vi "ReadTriggerNode.vi"(8 "Error In":errorcluster, 11 "Multiplexer Node In":refnum<k20>) -> (0 "Error Out":errorcluster, 2 "Trigger Configuration":T1={"Arm"={"Source"=enum."Hold", "Count"=1, "Infinite?"=FALSE}, "Scan"={"Source"=enum."Hold", "Count"=0, "Infinite?"=FALSE, "Delay (sec)"=0.0, "Interval (sec)"=0.0}, "Channel"={"Source"=enum."Hold", "Count"=0, "Infinite?"=FALSE, "Auto Count?"=FALSE, "Delay (sec)"=0.0, "Interval (sec)"=0.0}} {"Arm"."Count" min=1 max=99999 step=1}, 3 "Multiplexer Node Out":refnum<k20>)   [LabVIEW 2012]
uses:
  TriggerConfiguration.ctl
  TriggerArmConfiguration.ctl
  driver/Public/Controls/ArmSource.ctl
  TriggerScanConfiguration.ctl
  driver/Public/Controls/ScanSource.ctl
  TriggerChannelConfiguration.ctl
  driver/Public/Controls/TriggerSource.ctl
  driver/Keithley-7001.lvlib
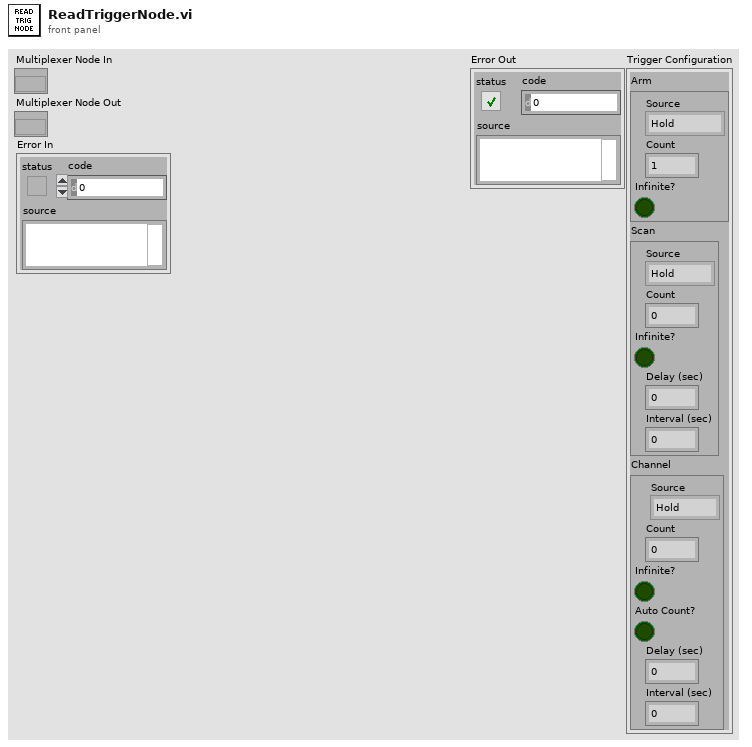
[diagram p1: front panel]
types:
  T1 = typedef "TriggerConfiguration.ctl" = cluster{"Arm":T2, "Scan":T4, "Channel":T6}
  T2 = typedef "TriggerArmConfiguration.ctl" = cluster{"Source":T3, "Count":u32, "Infinite?":bool}
  T3 = typedef "Keithley-7001.lvlib/ArmSource.ctl" = enum16{"Hold", "Immediate", "Manual", "Bus", "TLink", "External"}
  T4 = typedef "TriggerScanConfiguration.ctl" = cluster{"Source":T5, "Count":u32, "Infinite?":bool, "Delay (sec)":dbl, "Interval (sec)":dbl}
  T5 = typedef "Keithley-7001.lvlib/ScanSource.ctl" = enum16{"Hold", "Immediate", "Timer", "Manual", "Bus", "TLink", "External"}
  T6 = typedef "TriggerChannelConfiguration.ctl" = cluster{"Source":T7, "Count":u32, "Infinite?":bool, "Auto Count?":bool, "Delay (sec)":dbl, "Interval (sec)":dbl}
  T7 = typedef "Keithley-7001.lvlib/TriggerSource.ctl" = enum16{"Hold", "Immediate", "Manual", "Bus", "TLink", "External", "Timer"}
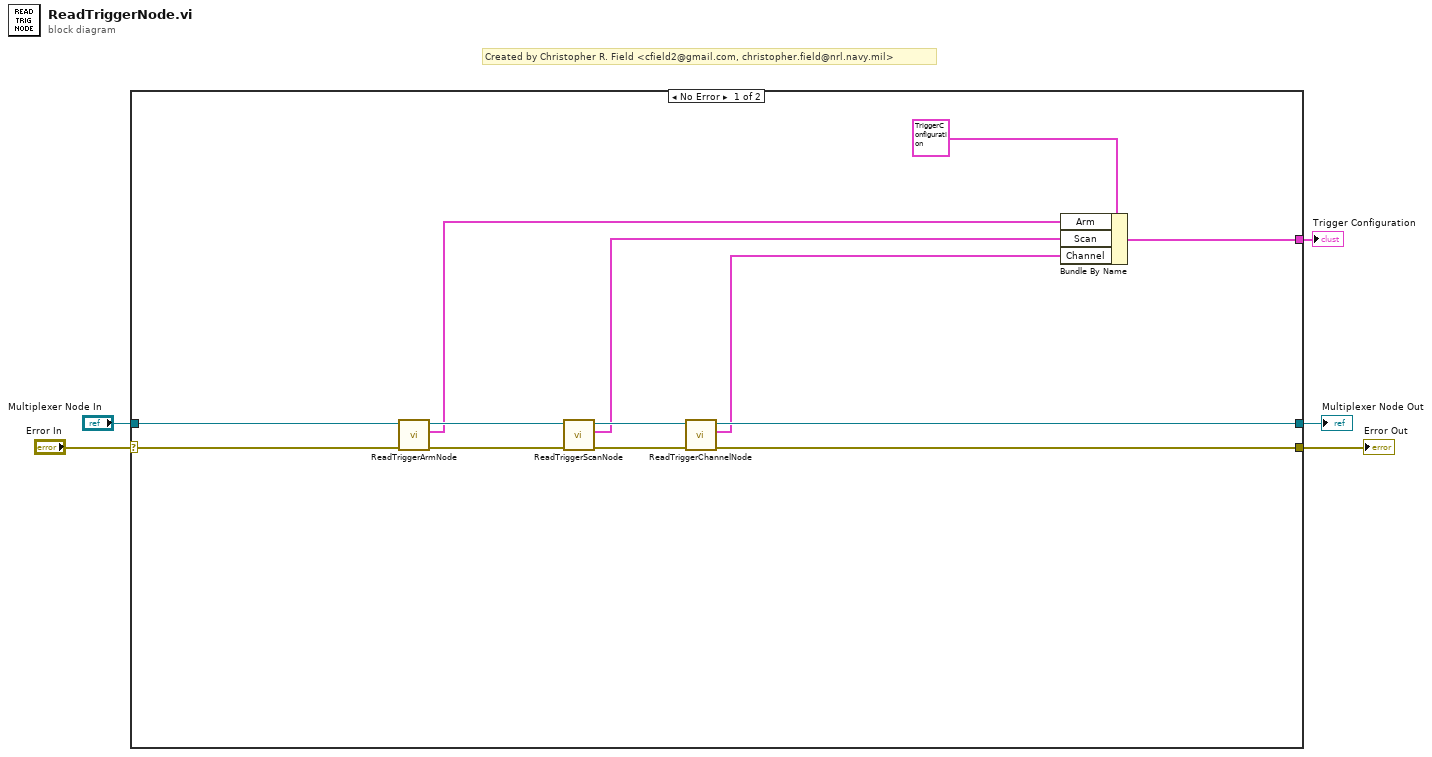
[diagram p0: block diagram]
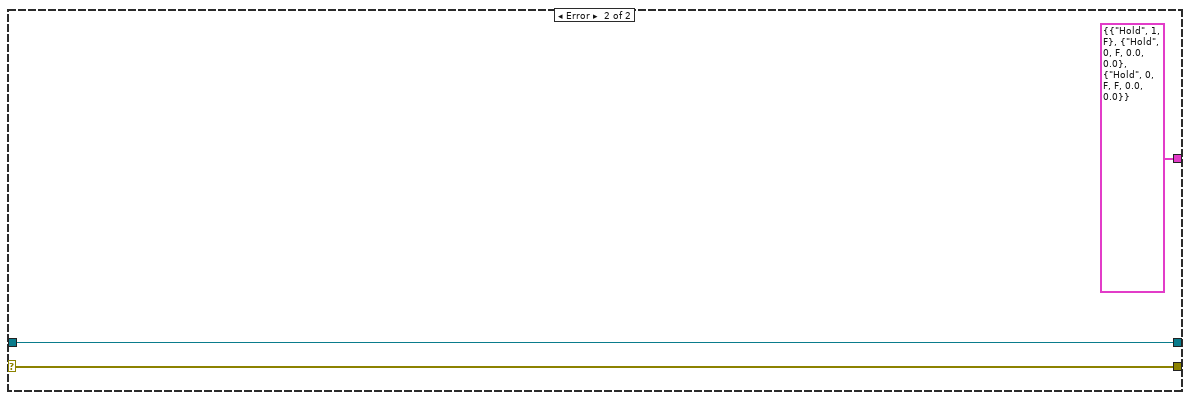
[diagram p2: hidden frame]
diagram:
  # "Created by Christopher R. Field <cfield2@gmail.com, christopher.field@nrl.navy.mil>"
  n1 = case shown="No Error" "Error In" {
    selector: "Error In" -> [w11 w19]
    tunnel: "Multiplexer Node In" -> [w14 w20]
    tunnel: [w13 w20] -> w4
    tunnel: [w12 w19] -> w3
    tunnel: [w6 T1 {"Arm"={"Source"=enum."Hold", "Count"=1, "Infinite?"=FALSE}, "Scan"={"Source"=enum."Hold", "Count"=0, "Infinite?"=FALSE, "Delay (sec)"=0.0, "Interval (sec)"=0.0}, "Channel"={"Source"=enum."Hold", "Count"=0, "Infinite?"=FALSE, "Auto Count?"=FALSE, "Delay (sec)"=0.0, "Interval (sec)"=0.0}} ("Trigger Configuration")] -> w1
    frame No Error {
      n2 = call "ReadTriggerArmNode.vi"("Error In"=w11, "Multiplexer Node In"=w14) -> ("Error Out"=w15:errorcluster, "Trigger Arm Configuration"=w9:T2, "Multiplexer Node Out"=w18:refnum<k20>)  [unwired: 7 in]
      n3 = call "ReadTriggerScanNode.vi"("Error In"=w15, "Multiplexer Node In"=w18) -> ("Error Out"=w16:errorcluster, "Trigger Scan Configuration"=w8:T4, "Multiplexer Node Out"=w17:refnum<k20>)  [unwired: 7 in]
      n4 = call "ReadTriggerChannelNode.vi"("Error In"=w16, "Multiplexer Node In"=w17) -> ("Error Out"=w12:errorcluster, "Trigger Channel Configuration"=w7:T6, "Multiplexer Node Out"=w13:refnum<k20>)  [unwired: 7 in]
      n5 = Bundle By Name(cluster=T1 {"Arm"={"Source"=enum."Hold", "Count"=1, "Infinite?"=FALSE}, "Scan"={"Source"=enum."Hold", "Count"=0, "Infinite?"=FALSE, "Delay (sec)"=0.0, "Interval (sec)"=0.0}, "Channel"={"Source"=enum."Hold", "Count"=0, "Infinite?"=FALSE, "Auto Count?"=FALSE, "Delay (sec)"=0.0, "Interval (sec)"=0.0}} ("Trigger Configuration"), "Arm"=w9, "Scan"=w8, "Channel"=w7) -> (w6:T1)
    }
    frame Error {
    }
  }
  "Multiplexer Node Out" <- w4
  "Error Out" <- w3
  "Trigger Configuration" <- w1
